vi "CheckUserValidation.vi"() -> ()   [LabVIEW 2024]
uses:
  <vilib>/addons/database/Auxilliary.llb/DB Tools Cursor Type.ctl
  <vilib>/addons/database/Connection.llb/DB Tools Open Connec (Path).vi
  <vilib>/addons/database/Connection.llb/Conn Execute.vi
  <vilib>/addons/database/Recordset.llb/Rec Fetch Recordset Data (R).vi
  <vilib>/addons/database/Recordset.llb/Rec Destroy - Connection.vi
  <vilib>/addons/database/NI_Database_API.lvlib
panel:
  out "recordset data":variant[][](array[variant])
  out "String":string
  in  "Password":string
  in  "UserName":string
  out "error out":errorcluster
  in  "error in":errorcluster
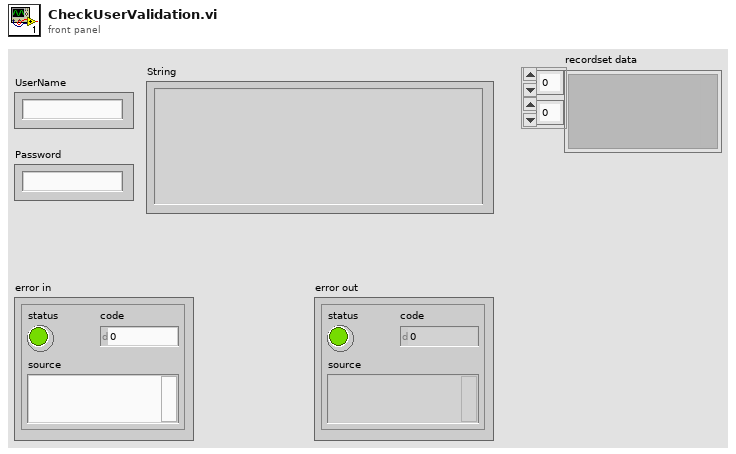
[diagram p1: front panel]
types:
  T1 = typedef "NI_Database_API.lvlib/DB Tools Cursor Type.ctl" = enum16{"forward-only", "keyset", "dynamic", "static"}
  T2 = typedef "NI_Database_API.lvlib/Conn ObjectReference.ctl" = refnum<k1>
  T3 = typedef "NI_Database_API.lvlib/Rec ObjectReference.ctl" = refnum<k1>
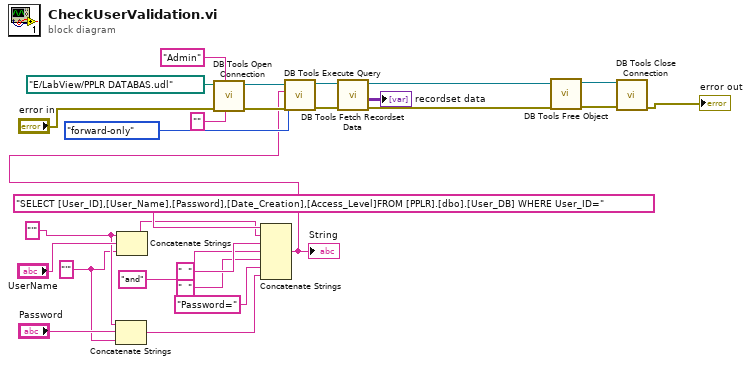
[diagram p0: block diagram]
diagram:
  w16 = "'"
  w18 = "'"
  n1 = Concatenate Strings(w18, "Password", w16) -> (w10:string)
  n2 = Concatenate Strings(w18, "UserName", w16) -> (w15:string)
  n3 = call-poly <vilib>:"DB Tools Open Connection.vi"("password"="", "userID"="Admin", "error in (no error)"="error in", "connection information"=path "E:/LabView/PPLR DATABAS.udl") -> ("error out"=w22:errorcluster, "connection reference"=w23:T2)  [unwired: 4 in]
  n4 = Concatenate Strings("SELECT [User_ID],[User_Name],[Password],[Date_Creation],[Access_Level]FROM [PPLR].[dbo].[User_DB] WHERE User_ID=", w15, "  " ("string"), "and" ("string"), "  " ("string"), "Password=" ("string"), w10) -> (w9:string)
  "String" <- w9
  n5 = call-poly <vilib>:"DB Tools Execute Query.vi"("error in (no error)"=w22, "cursor type"=DB_Tools_Cursor_Type."forward-only", "SQL query"=w9, "connection reference"=w23) -> ("error out"=w7:errorcluster, "recordset reference"=w8:T3)  [unwired: 4 in]
  n6 = call-poly <vilib>:"DB Tools Fetch Recordset Data.vi"("error in (no error)"=w7, "recordset reference"=w8) -> ("error out"=w2:errorcluster, "recordset data"=→"recordset data":variant[][], "recordset reference out"=w3:T3)  [unwired: 3 in]
  n7 = call-poly <vilib>:"DB Tools Free Object.vi"("error in (no error)"=w2, "recordset reference"=w3) -> ("error out"=w5:errorcluster, "connection reference"=w6:T2)  [unwired: 8 in]
  n8 = call <vilib>:"DB Tools Close Connection.vi"("error in (no error)"=w5, "connection reference"=w6) -> ("error out"=→"error out":errorcluster)  [unwired: 5 in]
